vi "Wipe UI History.vi"(5 "Secondary Chart":refnum<vi>, 7 "Primary Chart":refnum<vi>, 8 "Error in":errorcluster, 11 "State Variables in":T1) -> (0 "error out":errorcluster, 3 "State Variables out":T1)   [LabVIEW 2014, in "Flow Control.lvlib"]
uses:
  Flow Control.lvlib
  Controls/State Variables.ctl
  Controls/DAQmx Variables.ctl
  Controls/Filter Variables.ctl
  Filter.lvlib
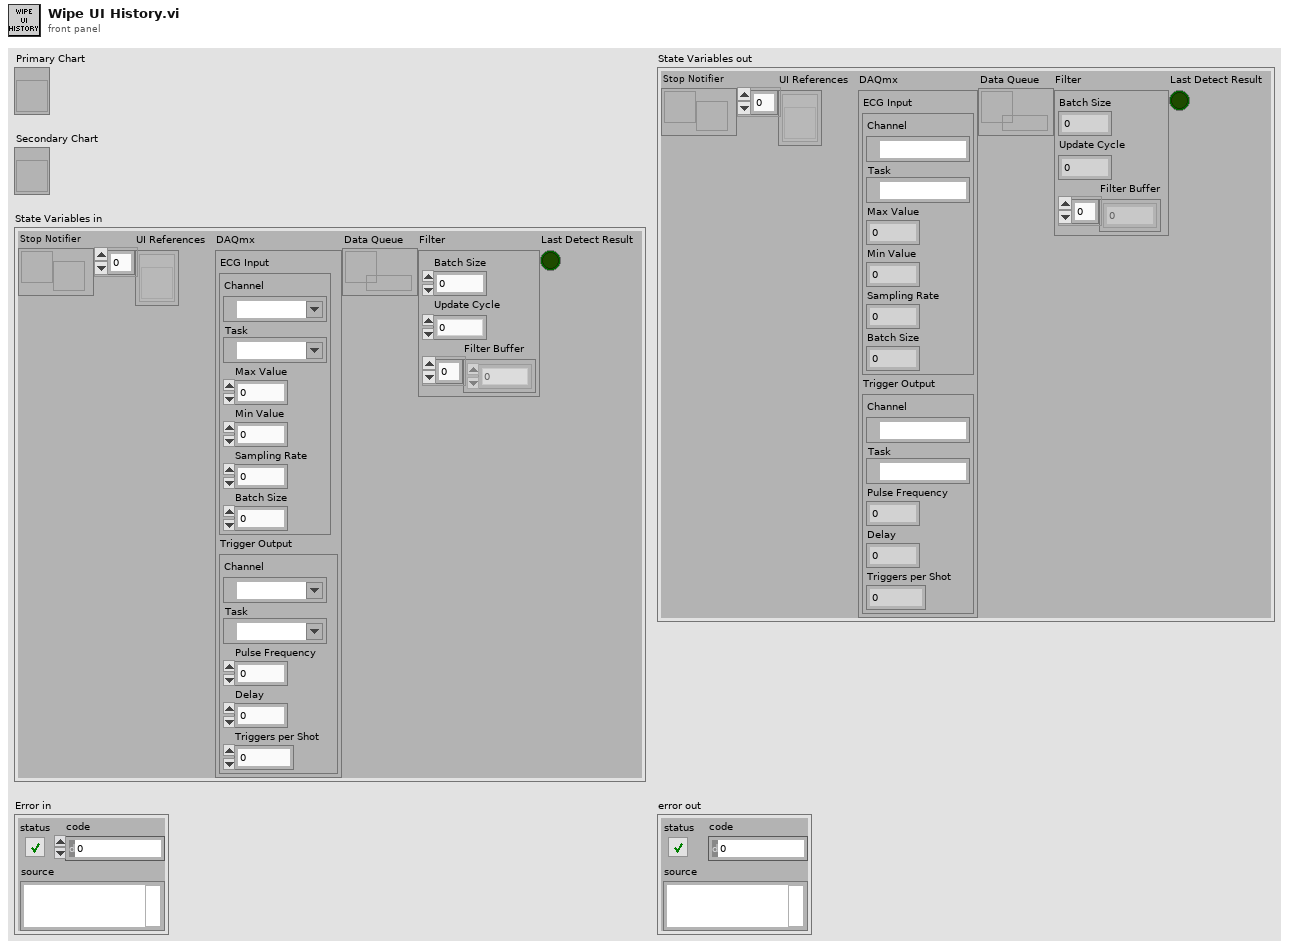
[diagram p1: front panel]
types:
  T1 = typedef "State Variables.ctl" = cluster{"Stop Notifier":refnum<notifier>, "UI References":refnum<vi>[], "DAQmx":T2, "Data Queue":refnum<queue>, "Filter":T3, "Last Detect Result":bool}
  T2 = typedef "DAQmx Variables.ctl" = cluster{"ECG Input":cluster{"Channel":tag, "Task":refnum<k21>, "Max Value":dbl, "Min Value":dbl, "Sampling Rate":dbl, "Batch Size":i32}, "Trigger Output":cluster{"Channel":tag, "Task":refnum<k21>, "Pulse Frequency":dbl, "Delay":u16, "Triggers per Shot":i32}}
  T3 = typedef "Filter Variables.ctl" = cluster{"Batch Size":i32, "Update Cycle":i32, "Filter Buffer":dbl[]}
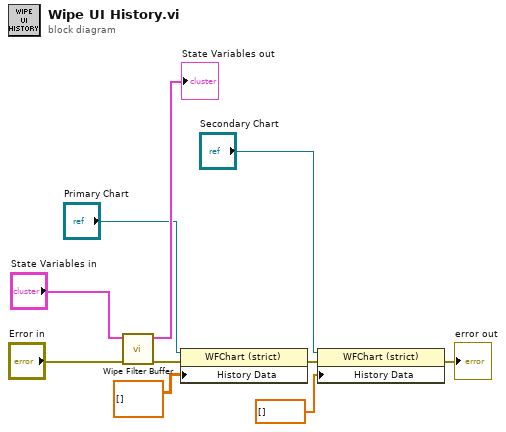
[diagram p0: block diagram]
diagram:
  n1 = call "Wipe Filter Buffer.vi"("Error in"="Error in", "State Variables in"="State Variables in") -> ("Error out"=w9:errorcluster, "State Variables out"=→"State Variables out":T1)  [unwired: 8 in]
  n2 = property on="Property Node" class="WFChart (strict)"(reference="Primary Chart", error in=w9, "History Data"=dbl[][] [] ("Signal Viewer")) -> (error out=w5:errorcluster)  [unwired: 1 out]
  n3 = property on="Property Node" class="WFChart (strict)"(reference="Secondary Chart", error in=w5, "History Data"=dbl[] []) -> (error out=→"error out":errorcluster)  [unwired: 1 out]
